vi "object detector (img as src).vi"() -> ()   [LabVIEW 2020]
uses:
  <vilib>/vision/Deep Learning.llb/IMAQ DL Model Type.ctl
  <vilib>/vision/Deep Learning.llb/IMAQ DL Model Objects.ctl
  <vilib>/vision/Deep Learning.llb/IMAQ DL Model Label.ctl
  <vilib>/vision/Deep Learning.llb/IMAQ DL Model Detect Objects Node Names.ctl
  <vilib>/vision/NI_Vision_Development_Module.lvlib
panel:
  in  "Метки":T1[](array[typedef])=[{"ID"=1, "Label"="airplane"}]
  out "Обнаруженные объекты":T2[](array[typedef]) {"Bounding Box"."y" format="%.2f"; "Bounding Box"."x" format="%.2f"}
  out "Image":T3(plugin-control)
  in  "Выбор изображения":i32
  in  "Stop":bool
  in  "Минимальный порог оценки":sgl=0.70000005 min=0 max=1 step=0.1 format="%.3g"
  in  "Каталог с тестовыми изображениями":path
  in  "Тип цвета изображений":T4 items=["Grayscale (U8)", "Grayscale (I16)", "Grayscale (SGL)", "Complex (CSG)", "RGB (U32)", "HSL (U32)", "RGB (U64)", "Grayscale (U16)"]
  in  "Тип модели":T5 items=["Frozen Graph", "Saved Model"]
  in  "Граф":path
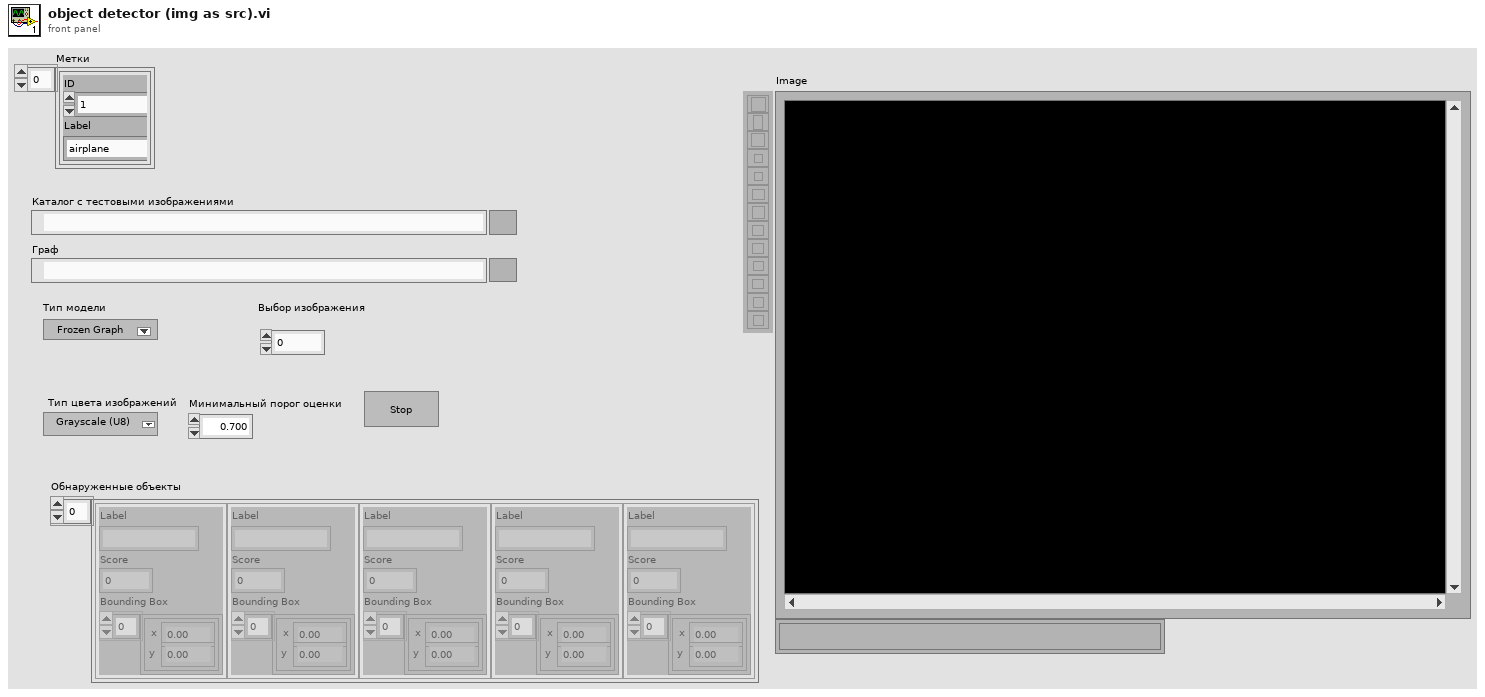
[diagram p1: front panel]
types:
  T1 = typedef "IMAQ DL Model Label.ctl" = cluster{"ID":u32, "Label":string}
  T2 = typedef "IMAQ DL Model Objects.ctl" = cluster{"Label":string, "Score":sgl, "Bounding Box":cluster{"x":sgl, "y":sgl}[]}
  T3 = typedef "IMAQ Image.ctl" = refnum<image>
  T4 = typedef "Image Type" = u32
  T5 = typedef "IMAQ DL Model Type.ctl" = i32
  T6 = typedef "IMAQ DL Model Refnum.ctl" = refnum<k20>
  T7 = typedef "IMAQ DL Model Detect Objects Node Names.ctl" = cluster{"Number of Objects":string, "Labels":string, "Scores":string, "Bounding Boxes":string}
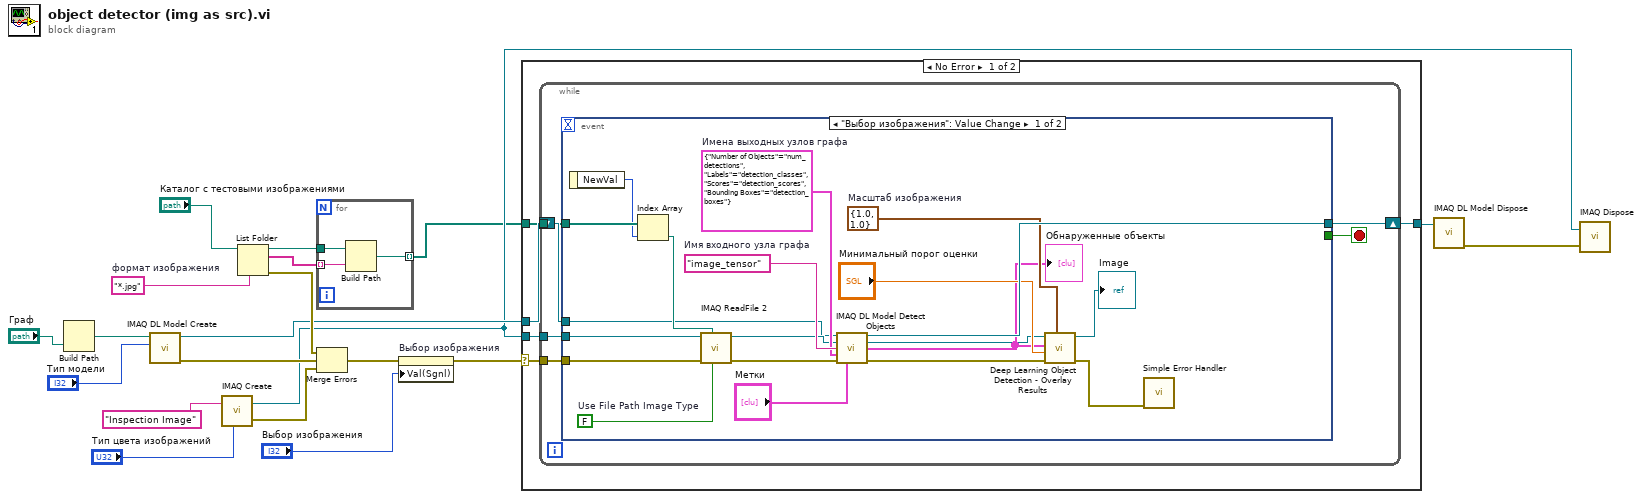
[diagram p0: block diagram]
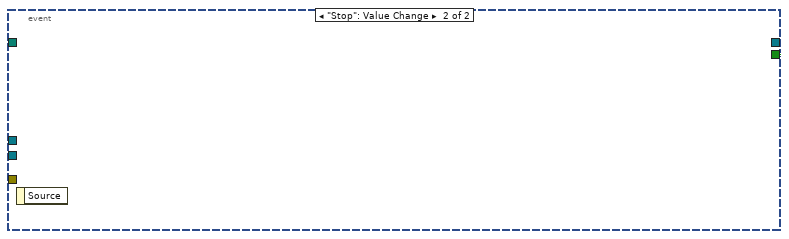
[diagram p2: hidden frame]
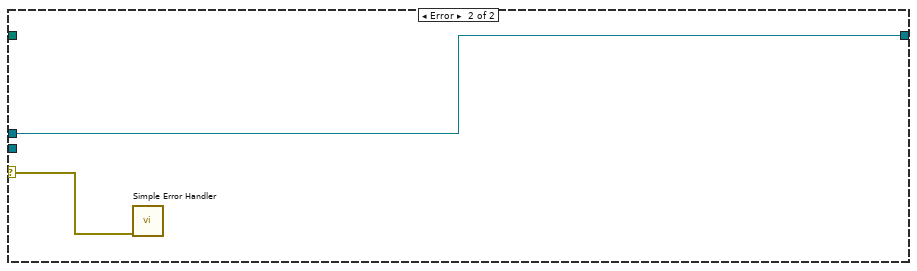
[diagram p3: hidden frame]
diagram:
  w1 = "*.jpg"  # формат изображения
  n1 = Build Path(name or relative path="Граф") -> (appended path=w18:path)  [unwired: 1 in]
  n2 = call-poly "IMAQ DL Model Create"("Model Type"="Тип модели", "File Path"=w18) -> ("error out"=w9:errorcluster, "Model Refnum"=w8:T6)  [unwired: 8 in]
  n3 = call "IMAQ Create"("Image Name"="Inspection Image", "Image Type"="Тип цвета изображений") -> ("New Image"=w7:T3, "error out"=w15:errorcluster)  [unwired: 3 in]
  n4 = List Folder(path="Каталог с тестовыми изображениями", pattern=w1) -> (path out=w17:path, filenames=w16:string[], error out=w14:errorcluster)  [unwired: 1 in, 2 out]
  n5 = for {
    tunnel: w17 -> [w23]
    tunnel: w16 -> [w22] mode=indexing
    tunnel: [w21] -> w4 mode=indexing
    n6 = Build Path(base path=w23, name or relative path=w22) -> (appended path=w21:path)
  }
  n7 = Merge Errors "Merge Errors"(w14, w9, w15) -> (w13:errorcluster)
  n8 = property on="Выбор изображения" class="DigNum (strict)"(error in=w13, "Val(Sgnl)"="Выбор изображения") -> (error out=w2:errorcluster)  [unwired: 1 in, 1 out]
  n9 = case shown="No Error" w2 {
    selector: w2 -> [w24 w56]
    tunnel: w8 -> [w28 w57]
    tunnel: w7 -> [w27 _]
    tunnel: w4 -> [w26 _]
    tunnel: [w25 w57] -> w3
    frame No Error {
      n10 = while {
        shift-right: [w32] -> w25
        shift-left: w28 -> [w34]
        tunnel: w26 -> [w31]
        tunnel: w27 -> [w30]
        tunnel: w24 -> [w29]
        stop <- w33 stop-if-true
        n11 = event shown="[0] \"Выбор изображения\": Value Change" {
          selector: _ -> [_ _]
          dyn-events: _ -> [_ _]
          timeout: _ -> [_ _]
          tunnel: w34 -> [w35 _]
          tunnel: [_ "Stop"] -> w33
          tunnel: [w54 _] -> w32
          tunnel: w31 -> [w51 _]
          tunnel: w30 -> [w49 _]
          tunnel: w29 -> [w46 _]
          event "Выбор изображения": Value Change {
            w40 = FALSE  # Use File Path Image Type
            w44 = T7 {"Number of Objects"="num_detections", "Labels"="detection_classes", "Scores"="detection_scores", "Bounding Boxes"="detection_boxes"}  # Имена выходных узлов графа
            w45 = "image_tensor"  # Имя входного узла графа
            w48 = cluster{"X":dbl, "Y":dbl} {"X"=1.0, "Y"=1.0}  # Масштаб изображения
            n12 = event-data() -> ("NewVal"=w42:i32)  [unwired: 1 in]
            n13 = Index Array "Index Array"(array=w51, index=w42) -> (element=w50:path)
            n14 = call "IMAQ ReadFile 2"("Use File Path Image Type"=w40, "File Path"=w50, "error in (no error)"=w46, "Image"=w49) -> ("error out"=w37:errorcluster, "Image Out"=w38:T3)  [unwired: 3 in, 3 out]
            n15 = call "IMAQ DL Model Detect Objects"("Model Refnum In"=w35, "Image"=w38, "Input Node Name"=w45, "Output Node Names"=w44, "error in (no error)"=w37, "Labels"="Метки") -> ("Model Refnum Out"=w54:T6, "Image (duplicate)"=w47:T3, "Detected Objects"=w43:T2[], "error out"=w52:errorcluster)  [unwired: 5 in, 1 out]
            "Обнаруженные объекты" <- w43
            n16 = call "Deep Learning Object Detection - Overlay Results.vi"("Image Scaling"=w48, "error in (no error)"=w52, "Minimum Score Threshold"="Минимальный порог оценки", "Detected Objects"=w43, "Image In"=w47) -> ("error out"=w41:errorcluster, "Image Out"=→"Image":T3)  [unwired: 5 in]
            n17 = call <vilib>:"Simple Error Handler.vi"("error in (no error)"=w41) -> ()  [unwired: 4 in, 5 out]
          }
          event "Stop": Value Change {
            n18 = event-data() -> ()  [unwired: 1 in, 1 out]
          }
        }
      }
    }
    frame Error {
      n19 = call <vilib>:"Simple Error Handler.vi"("error in (no error)"=w56) -> ()  [unwired: 4 in, 5 out]
    }
  }
  n20 = call "IMAQ DL Model Dispose"("Model Refnum"=w3) -> ("error out"=w11:errorcluster)  [unwired: 10 in]
  n21 = call "IMAQ Dispose"("Image"=w7, "error in (no error)"=w11) -> ()  [unwired: 4 in, 1 out]
